vi "Call Stack to String.vi"(10 "With EOL Separator":bool, 11 "Call Stacks to Skip":i32=2) -> (3 "Call Stack String":string)   [LabVIEW 2014, in "Robot Actor Framework.lvlib" / "Utilities.lvlib"]
uses:
  Utilities.lvlib
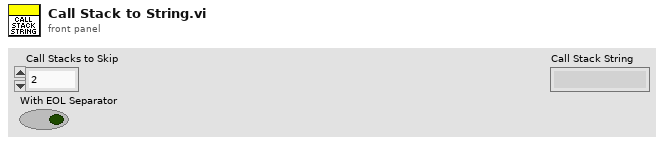
[diagram p1: front panel]
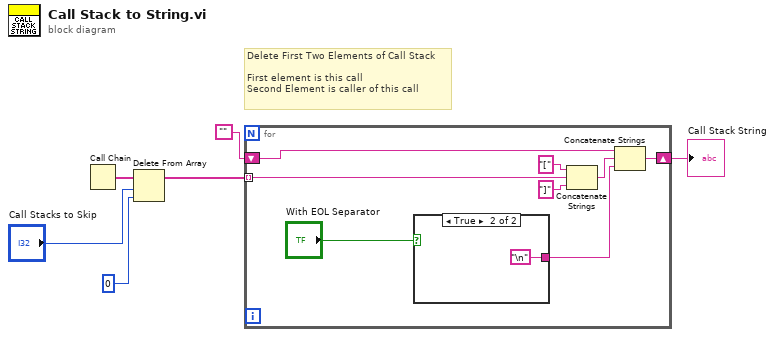
[diagram p0: block diagram]
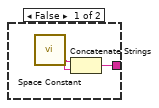
[diagram p2: hidden frame]
diagram:
  # "Delete First Two Elements of Call Stack\n\nFirst element is this call\nSecond Element is caller of this call"
  n1 = Call Chain() -> (call chain=w6:string[])
  n2 = Delete From Array "Delete From Array"(array=w6, length="Call Stacks to Skip", index=0) -> (array with subset deleted=w2:string[])  [unwired: 1 out]
  n3 = for {
    tunnel: w2 -> [w12] mode=indexing
    shift-right: [w14] -> w1
    shift-left: "" -> [w13]
    n4 = case shown="True" "With EOL Separator" {
      tunnel: [w15 "\n"] -> w7
      frame False {
        n5 = call <vilib>:"Space Constant.vi"() -> ("String"=w16:string)
        n6 = Concatenate Strings(w16, w16) -> (w15:string)
      }
      frame True {
      }
    }
    n7 = Concatenate Strings("[" ("string"), w12, "]" ("string")) -> (w10:string)
    n8 = Concatenate Strings(w13, w10, w7) -> (w14:string)
  }
  "Call Stack String" <- w1
